vi "Configure Camera Setting.vi"(4 "lower limit":i64=-1000000, 6 "upper limit":i64=1000000, 8 "Desired Value":string, 9 "Mode":string, 10 "Desired Value":i64, 11 "Session In":T1) -> (2 "Set Value":i64, 3 "Session out":T1)   [LabVIEW 2015]
uses:
  <vilib>/userdefined/High Color/IMAQdx.ctl
  <resource>/objmgr/imaqdx.rc
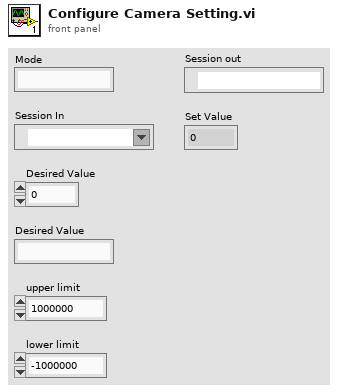
[diagram p1: front panel]
types:
  T1 = typedef "IMAQdx.ctl" = refnum<k21>
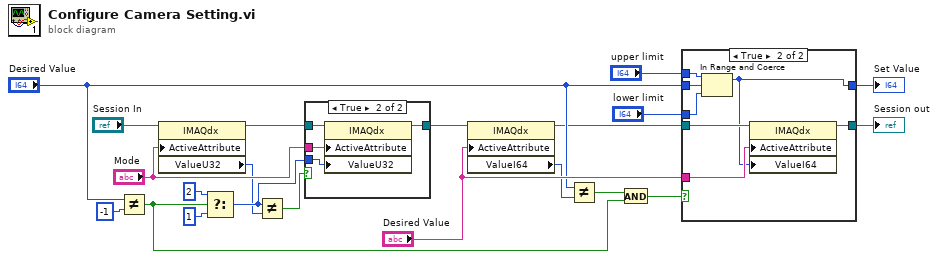
[diagram p0: block diagram]
diagram:
  n1 = Not Equal?(x="Desired Value", y=i64 -1) -> (x != y?=w11:bool)
  n2 = property class="IMAQdx"(reference="Session In", "ActiveAttribute"="Mode") -> (reference out=w7:T1, "ValueU32"=w4:u32)  [unwired: 1 in, 1 out]
  n3 = Select(t=u32 2 ("ValueU32"), s=w11, f=u32 1) -> (s? t:f=w6:u32)
  n4 = Not Equal?(x=w6, y=w4) -> (x != y?=w5:bool)
  n5 = case shown="True" w5 {
    tunnel: w6 -> [_ w26]
    tunnel: w7 -> [w22 w25]
    tunnel: [w22 w24] -> w8
    tunnel: "Mode" -> [_ w23]
    frame False {
    }
    frame True {
      n6 = property class="IMAQdx"(reference=w25, "ActiveAttribute"=w23, "ValueU32"=w26) -> (reference out=w24:T1)  [unwired: 1 in, 1 out]
    }
  }
  n7 = property class="IMAQdx"(reference=w8, "ActiveAttribute"="Desired Value") -> (reference out=w13:T1, "ValueI64"=w9:i64)  [unwired: 1 in, 1 out]
  n8 = Not Equal?(x="Desired Value", y=w9) -> (x != y?=w10:bool)
  n9 = And(x=w10, y=w11) -> (x .and. y?=w12:bool)
  n10 = case shown="True" w12 {
    tunnel: w13 -> [w28 w35]
    tunnel: "Desired Value" -> [w27 w32]
    tunnel: "Desired Value" -> [_ w34]
    tunnel: [w28 w33] -> w17
    tunnel: "upper limit" -> [_ w31]
    tunnel: "lower limit" -> [_ w30]
    tunnel: [w27 w29] -> w21
    frame False {
    }
    frame True {
      n11 = In Range and Coerce(upper limit=w31, x=w32, lower limit=w30) -> (coerced(x)=w29:i64)  [unwired: 1 out]
      n12 = property class="IMAQdx"(reference=w35, "ActiveAttribute"=w34, "ValueI64"=w29) -> (reference out=w33:T1)  [unwired: 1 in, 1 out]
    }
  }
  "Set Value" <- w21
  "Session out" <- w17
